vi "Dialogue_visa_TC1100_Emballage_BDD.vi"(6 "entrée d'erreur (pas d'erreur)":errorcluster, 9 "nom de ressource VISA":refnum<visa-resource-name>="ASRL3::INSTR") -> (0 "error out":errorcluster, 3 "buffer lu":string)   [LabVIEW 2020]
uses:
  Modules/FS/60_FS_Controles/60_FS_SetGet.ctl
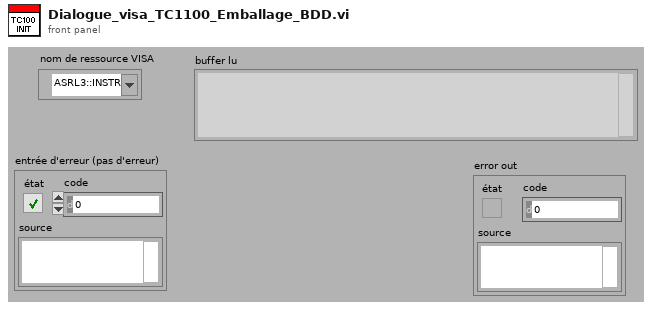
[diagram p1: front panel]
types:
  T1 = typedef "60_FS_SetGet.ctl" = enum16{"set", "get"}
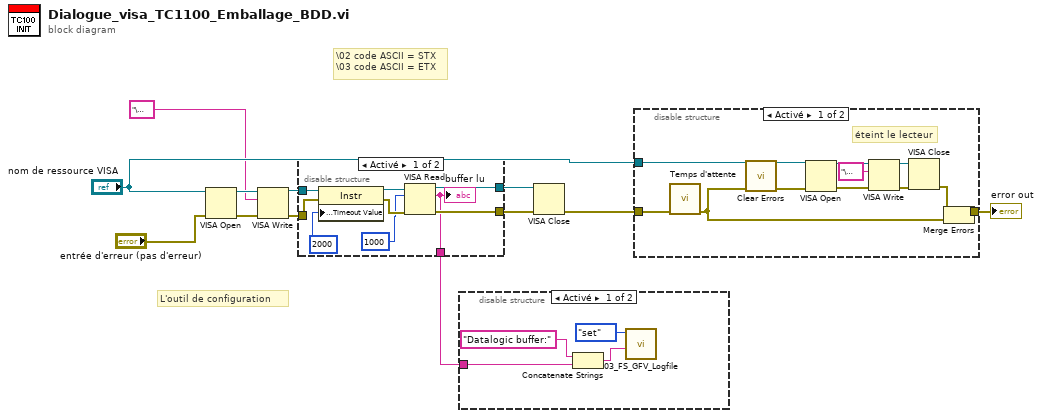
[diagram p0: block diagram]
diagram:
  # "L'outil de configuration"
  # "\\02 code ASCII = STX\n\\03 code ASCII = ETX"
  n1 = VISA Open(error in (no error)="entrée d'erreur (pas d'erreur)", VISA resource name="nom de ressource VISA") -> (VISA resource name=w11:refnum<visa-resource-name>, error out=w12:errorcluster)  [unwired: 3 in]
  n2 = VISA Write(VISA resource name=w11, write buffer="\u0002", error in (no error)=w12) -> (VISA resource name out=w9:refnum<visa-resource-name>, error out=w10:errorcluster)  [unwired: 1 out]
  n3 = disable-structure shown="Activé" {
    disable-tunnel: w10 -> [w21 w22]
    disable-tunnel: w9 -> [w20 w23]
    disable-tunnel: [w17 w22] -> w8
    disable-tunnel: [w16 w23] -> w7
    disable-tunnel: [w13 _] -> w1
    frame Enabled {
      n4 = property class="Instr"(reference=w20, error in=w21, "General Settings:Timeout Value"=u32 2000 ("Tmo Value")) -> (reference out=w18:refnum<visa-resource-name>, error out=w19:errorcluster)
      n5 = VISA Read(VISA resource name=w18, byte count=u32 1000 ("byte count (0)"), error in (no error)=w19) -> (VISA resource name out=w16:refnum<visa-resource-name>, read buffer=w13:string, error out=w17:errorcluster)  [unwired: 1 out]
      "buffer lu" <- w13
    }
    frame Disabled {
    }
  }
  n6 = disable-structure shown="Activé" {
    disable-tunnel: w1 -> [w24 _]
    frame Enabled {
      n7 = Concatenate Strings("Datalogic buffer:" ("Chaîne"), w24) -> (w26:string)
      n8 = call "03_FS_GFV_Logfile.vi"("Chaîne"=w26, "States"=60_FS_SetGet."set") -> ()  [unwired: 8 in, 2 out]
    }
    frame Disabled {
    }
  }
  n9 = VISA Close(VISA resource name=w7, error in (no error)=w8) -> (error out=w5:errorcluster)
  n10 = disable-structure shown="Activé" {
    disable-tunnel: "nom de ressource VISA" -> [w33 _]
    disable-tunnel: w5 -> [w32 w39]
    disable-tunnel: [w30 w39] -> w4
    frame Enabled {
      # "éteint le lecteur"
      n11 = call "Temps d'attente"("error in (no error)"=w32) -> ("error out"=w29:errorcluster)  [unwired: 10 in]
      n12 = call <vilib>:"Clear Errors.vi"("error in (no error)"=w29) -> ("error out"=w28:errorcluster)  [unwired: 5 in, 1 out]
      n13 = VISA Open(error in (no error)=w28, VISA resource name=w33) -> (VISA resource name=w35:refnum<visa-resource-name>, error out=w37:errorcluster)  [unwired: 3 in]
      n14 = VISA Write(VISA resource name=w35, write buffer="\u0003", error in (no error)=w37) -> (VISA resource name out=w34:refnum<visa-resource-name>, error out=w36:errorcluster)  [unwired: 1 out]
      n15 = VISA Close(VISA resource name=w34, error in (no error)=w36) -> (error out=w31:errorcluster)
      n16 = Merge Errors(w31, w29) -> (w30:errorcluster)
    }
    frame Disabled {
    }
  }
  "error out" <- w4
